vi "fixTarget.vi"(4 "LastTarget":dbl[](array[numeric]), 6 "Robot":refnum<class "Robot.lvclass">, 8 "error in (no error)":errorcluster, 9 "Ball":refnum<class "Ball.lvclass">, 10 "Target in":dbl[](array[numeric]), 11 "KickToSkill in":refnum<class "KickToSkill.lvclass">) -> (0 "error out":errorcluster, 2 "Target out":dbl[](array[numeric]), 3 "KickToSkill out":refnum<class "KickToSkill.lvclass">)   [LabVIEW 2023, in "KickToSkill.lvclass"]
uses:
  KickToSkill.lvclass
  Robot_class/Robot.lvclass
  Ball_class/Ball.lvclass
  Utilities_class/Utilities.lvclass
  Object_class/Object.lvclass/Object.ctl
  Object_class/Read x.vi
  Object_class/Read y.vi
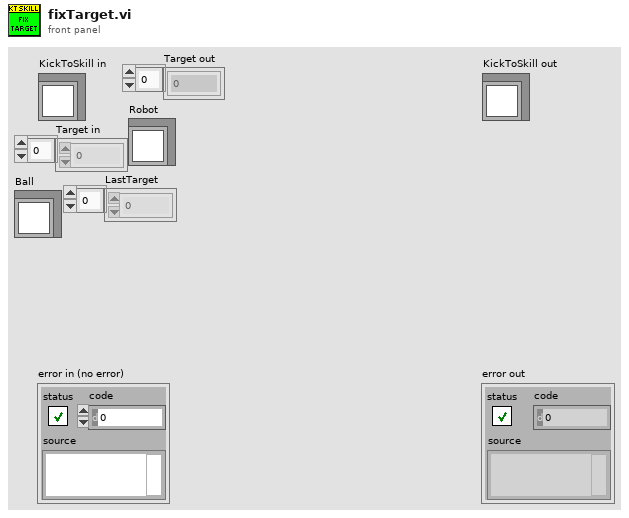
[diagram p1: front panel]
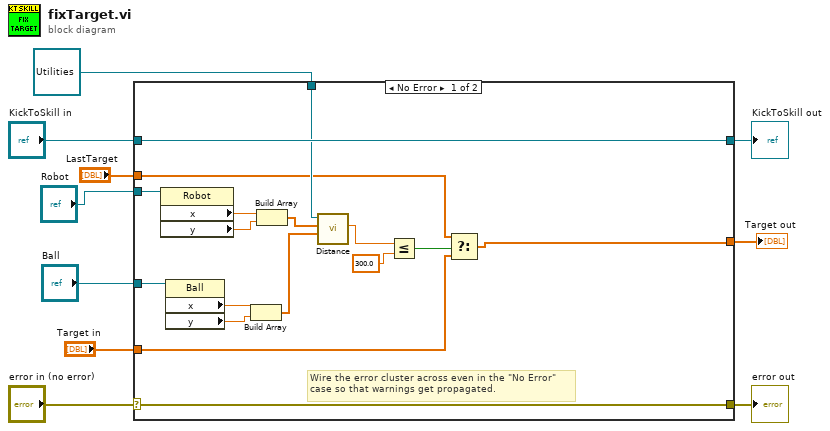
[diagram p0: block diagram]
diagram:
  n1 = case shown="No Error" "error in (no error)" {
    selector: "error in (no error)" -> [w26 w29]
    tunnel: [w26 w29] -> w9
    tunnel: [w27 w28] -> w7
    tunnel: "KickToSkill in" -> [w27 w28]
    tunnel: "Robot" -> [w25 _]
    tunnel: "Ball" -> [w24 _]
    tunnel: refnum<class "Utilities.lvclass"> refnum ("Utilities in") -> [w17 _]
    tunnel: "LastTarget" -> [w14 _]
    tunnel: "Target in" -> [w13 _]
    tunnel: [w12 _] -> w1
    frame No Error {
      # "Wire the error cluster across even in the \"No Error\"\ncase so that warnings get propagated."
      n2 = property class="Robot"(reference=w25) -> ("x"=w21:dbl, "y"=w20:dbl)  [unwired: 1 in, 2 out]
      n3 = property class="Ball"(reference=w24) -> ("x"=w23:dbl, "y"=w22:dbl)  [unwired: 1 in, 2 out]
      n4 = Build Array(w23, w22) -> (w18:dbl[])
      n5 = Build Array(w21, w20) -> (w19:dbl[])
      n6 = call-dynamic "Distance.vi"("P1"=w18, "P2"=w19, "Utilities in"=w17) -> ("Distance"=w16:dbl)  [unwired: 6 in, 2 out]
      n7 = Less Or Equal?(x=w16, y=300.0) -> (x <= y?=w11:bool)
      n8 = Select(t=w14, s=w11, f=w13) -> (s? t:f=w12:dbl[])
    }
    frame Error {
    }
  }
  "error out" <- w9
  "KickToSkill out" <- w7
  "Target out" <- w1
